vi "arm-lift-bang-bang-control.vi"(10 "PV Deg":dbl, 11 "SP DEG":dbl) -> (3 "CO Motor Out":dbl)   [LabVIEW 2019]
uses:
  <vilib>/Rock Robotics/WPI/ThirdParty/JAS_Junk/TrajLib/SlewRateLimiter_New.vi
  <vilib>/Rock Robotics/WPI/ThirdParty/JAS_Junk/TrajLib/SlewRateLimiter_Reset.vi
  <vilib>/Rock Robotics/WPI/ThirdParty/JAS_Junk/TrajLib/SlewRateLimiter_Calculate.vi
  <vilib>/Rock Robotics/WPI/ThirdParty/JAS_Junk/TrajLib/SlewRateLimiter_SetRate.vi
  <vilib>/Rock Robotics/WPI/ThirdParty/JAS_Junk/TrajLib/BangBang_AtSetpoint.vi
  <vilib>/Rock Robotics/WPI/ThirdParty/JAS_Junk/TrajLib/Util_GetTime.vi
  <vilib>/Rock Robotics/WPI/ThirdParty/JAS_Junk/TrajLib/VI/Util_GetTime_U32.vi
  <vilib>/Rock Robotics/WPI/ThirdParty/JAS_Junk/TrajLib/VI/Util_GetTime_U64.vi
  <vilib>/Rock Robotics/WPI/ThirdParty/JAS_Junk/TrajLib/BangBang_New.vi
  <vilib>/Rock Robotics/WPI/ThirdParty/JAS_Junk/TrajLib/BangBang_Calculate_SP_PV.vi
  <vilib>/Rock Robotics/WPI/ThirdParty/JAS_Junk/TrajLib/Trajectory_Library.lvlib
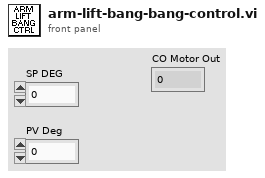
[diagram p1: front panel]
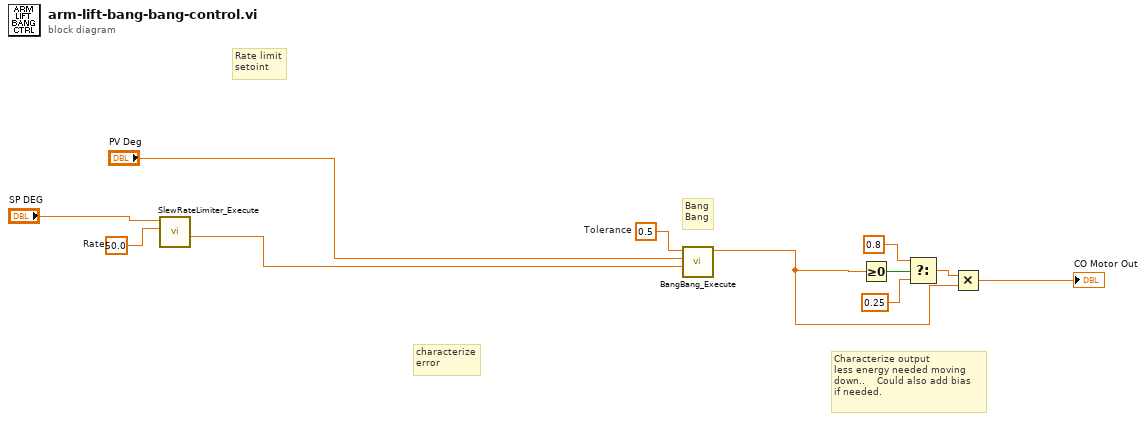
[diagram p0: block diagram]
diagram:
  w4 = 0.5  # Tolerance
  w5 = 50.0  # Rate
  # "Bang\nBang"
  # "Characterize output\nless energy needed moving\ndown..    Could also add bias\nif needed."
  # "Rate limit\nsetoint"
  # "characterize\nerror"
  n1 = call <vilib>:"SlewRateLimiter_Execute.vi"("PositiveRate"=w5, "Input"="SP DEG") -> ("Output"=w1:dbl)  [unwired: 8 in, 1 out]
  n2 = call <vilib>:"BangBang_Execute.vi"("Setpoint"=w1, "Measurment"="PV Deg", "Tolerance"=w4) -> ("ControlOutput"=w3:dbl)  [unwired: 6 in, 2 out]
  n3 = Greater Or Equal To 0?(x=w3) -> (x >= 0?=w6:bool)
  n4 = Select(t=0.8, s=w6, f=0.25) -> (s? t:f=w9:dbl)
  n5 = Multiply(x=w9, y=w3) -> (x*y=→"CO Motor Out":dbl)
